vi "发送组消息.vi"(7 "消息":string, 8 "错误输入（无错误）":errorcluster, 11 "队列组":T1) -> (0 "错误输出":errorcluster)   [LabVIEW 2021, in "QueueLib.lvlib"]
uses:
  QueueLib.lvlib
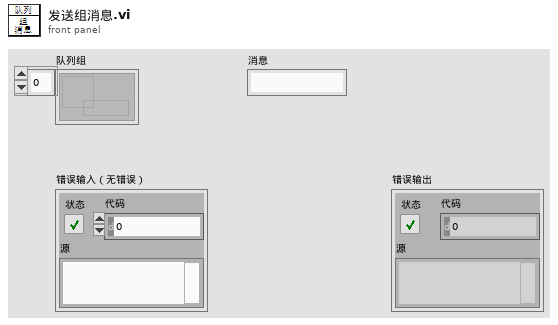
[diagram p1: front panel]
types:
  T1 = typedef "QueueLib.lvlib/队列组.ctl" = refnum<queue>[]
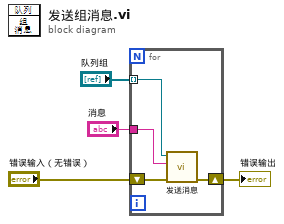
[diagram p0: block diagram]
diagram:
  n1 = for {
    tunnel: "队列组" -> [w7] mode=indexing
    tunnel: "消息" -> [w8]
    shift-right: [w6] -> w2
    shift-left: "错误输入（无错误）" -> [w5]
    n2 = call "发送消息.vi"("错误输入（无错误）"=w5, "消息"=w8, "输入队列"=w7) -> ("错误输出"=w6:errorcluster)  [unwired: 7 in, 1 out]
  }
  "错误输出" <- w2
